vi "System Configuration_Generator.vi"() -> ()   [LabVIEW 2020]
uses:
  LabVIEW 2020 Toolkits/VI Server Toolkit/VI Server_TypeDefs/VI Server_RefsCluster.ctl
  LabVIEW 2020 Toolkits/toolkits_lv2020_32bit/Synchronization.llb/SynchRefs_SetGet.ctl
  LabVIEW 2020 Toolkits/VI Server Toolkit/VI Server Libraries/VI Server_GetControl.llb/VI Server_1D_Array_STR_Get.vi
  LabVIEW 2020 Toolkits/VI Server Toolkit/VI Server Toolkit LV2013.lvlib
panel:
  in  "TabControls.SAVE":bool
  in  "TabControls.Name":string[](array[string])=["Tab.Main"] caption="Target VI: Tab Control Names"
  in  "VI.Server.Port":u32=3363 caption="VI Server Port"
  in  "SystemSettings.SAVE":bool caption="TabControls.SAVE"
  in  "SAVE":bool
  in  "Generate":bool caption="Generate [SET]"
  in  "Ind.Symbols":i32[](array[numeric])
  in  "Ctl.Symbols":i32[](array[numeric])
  out "#OfIndicators":i32 caption="# Of Indicators"
  in  "Tab.Main":enum32{"CONTROLS", "DATA", "INDICATORS"}(tab)
  in  "Controls":i32[](listbox)
  in  "[SET]":string
  in  "[GET] ARGUMENT 2":u16(ring) caption="[GET] ARGUMENT 2 Prototype" items=["AI.Averaged.Mesurement", "AI.ActualSampleRate", "AO.ActualSampleRate", "DI.Port.Lines.0:7", "DI.Port.Lines.8:15", "DI.Port.Lines.16:23", "DI.Port.Lines.24:31", "DI.Line.State", "DO.Line.State.Verify", "DO.Port.State.Verify", "**********************", "ctr0.In.Count", "ctr0.Out.Frequency.Actual", "ctr0.Out.Duty Cycle.Actual", "ctr1.In.Count", "ctr2.In.Count", "ctr3.In.Count", "ctr1.Out.Frequency.Actual", "ctr1.Out.Duty Cycle.Actual", "ctr2.Out.Frequency.Actual", "ctr2.Out.Duty Cycle.Actual", "ctr3.Out.Frequency.Actual", "ctr3.Out.Duty Cycle.Actual"]
  in  "[SET] ARGUMENT 2":u16(ring) caption="[SET] ARGUMENT 2 Prototype" items=["AI.Sample.Mode", "AI.TerminalConfiguration", "AI.MaxInputLimit", "AI.MinInputLimit", "AI.SampleRate", "AI.Number.Of.Samples", "AI.Measure", "AI.PhysicalChannel.Include", "AI.MultiChannelAcquisition", "**********************", "AO.Output", "AO.MinVoltage", "AO.MaxVoltage", "AO.SampleRate", "AO.NumberOfSamples", "AO.GenerationMode", "AO.SinewaveFrequency", "AO.SampleMode", "AO.Update", "**********************", "DI.Line.Update", "DI.Port.Update", "DO.Line.Update", "DO.Port.Lines.7:0", "DO.Port.Lines.15:8", "DO.Port.Lines.23:16", "DO.Port.Lines.31:24", "DO.Port.Update", "DO.Line.State", "DO.Port.Lines.7:0.Mask", "DO.Port.Lines.15:8.Mask", "DO.Port.Lines.23:16.Mask", "DO.Port.Lines.31:24.Mask", "DO.Port.Mask.Apply", "**********************", "Cntr.In.ActiveEdge", "Cntr.In.IntegrationTime", "Cntr.In.Start", "Cntr.Out.Frequency", "Cntr.Out.Duty.Cycle", "Cntr.Out.Sample.Mode", "Cntr.Out.Start", "Cntr.Out.NumberOfPulses", "Settings.LOAD", "Settings.Name.New"]
  in  "[Argument 3: Data Type]":string
  in  "[GET]":string
  in  "Indicators":i32[](listbox)
  in  "EXIT":bool
  in  "DataSource.FileType":i32(ring) caption="Data Source: FileType" items=["VI", "File: *.cfg"]
  out "#OfControls":i32 caption="# Of Controls"
  in  "SoftPanel.V.Load":bool caption="Data Source: Load"
  in  "SoftPanel.VI.Path":path caption="Soft Panel VI  Path"
  out "error out":errorcluster
  in  "error in":errorcluster
  # "INSTRUCTIONS:\n1. Select Soft Panel VI and press the button \"LOAD\".\n2. On the [CONTROLS] page, table \"Controls\", by double click, mark indicators which will be excluded from \nbeing included into a System Configuration.cfg file of the soft panel. \n3. On the [INDICTORS] page, table \"Indicators\", by double click mark indicators which will be excluded from \nbeing included into a System Configuration.cfg file of the soft panel.\n4. Press the \"GENERATE\" button and examine data in the [SET], [Argument3: data Type], and [GET] tables.\n5. Press the \"SAVE\" button to transfer data to the System Configuration.cfg file."
  # "System Settings"
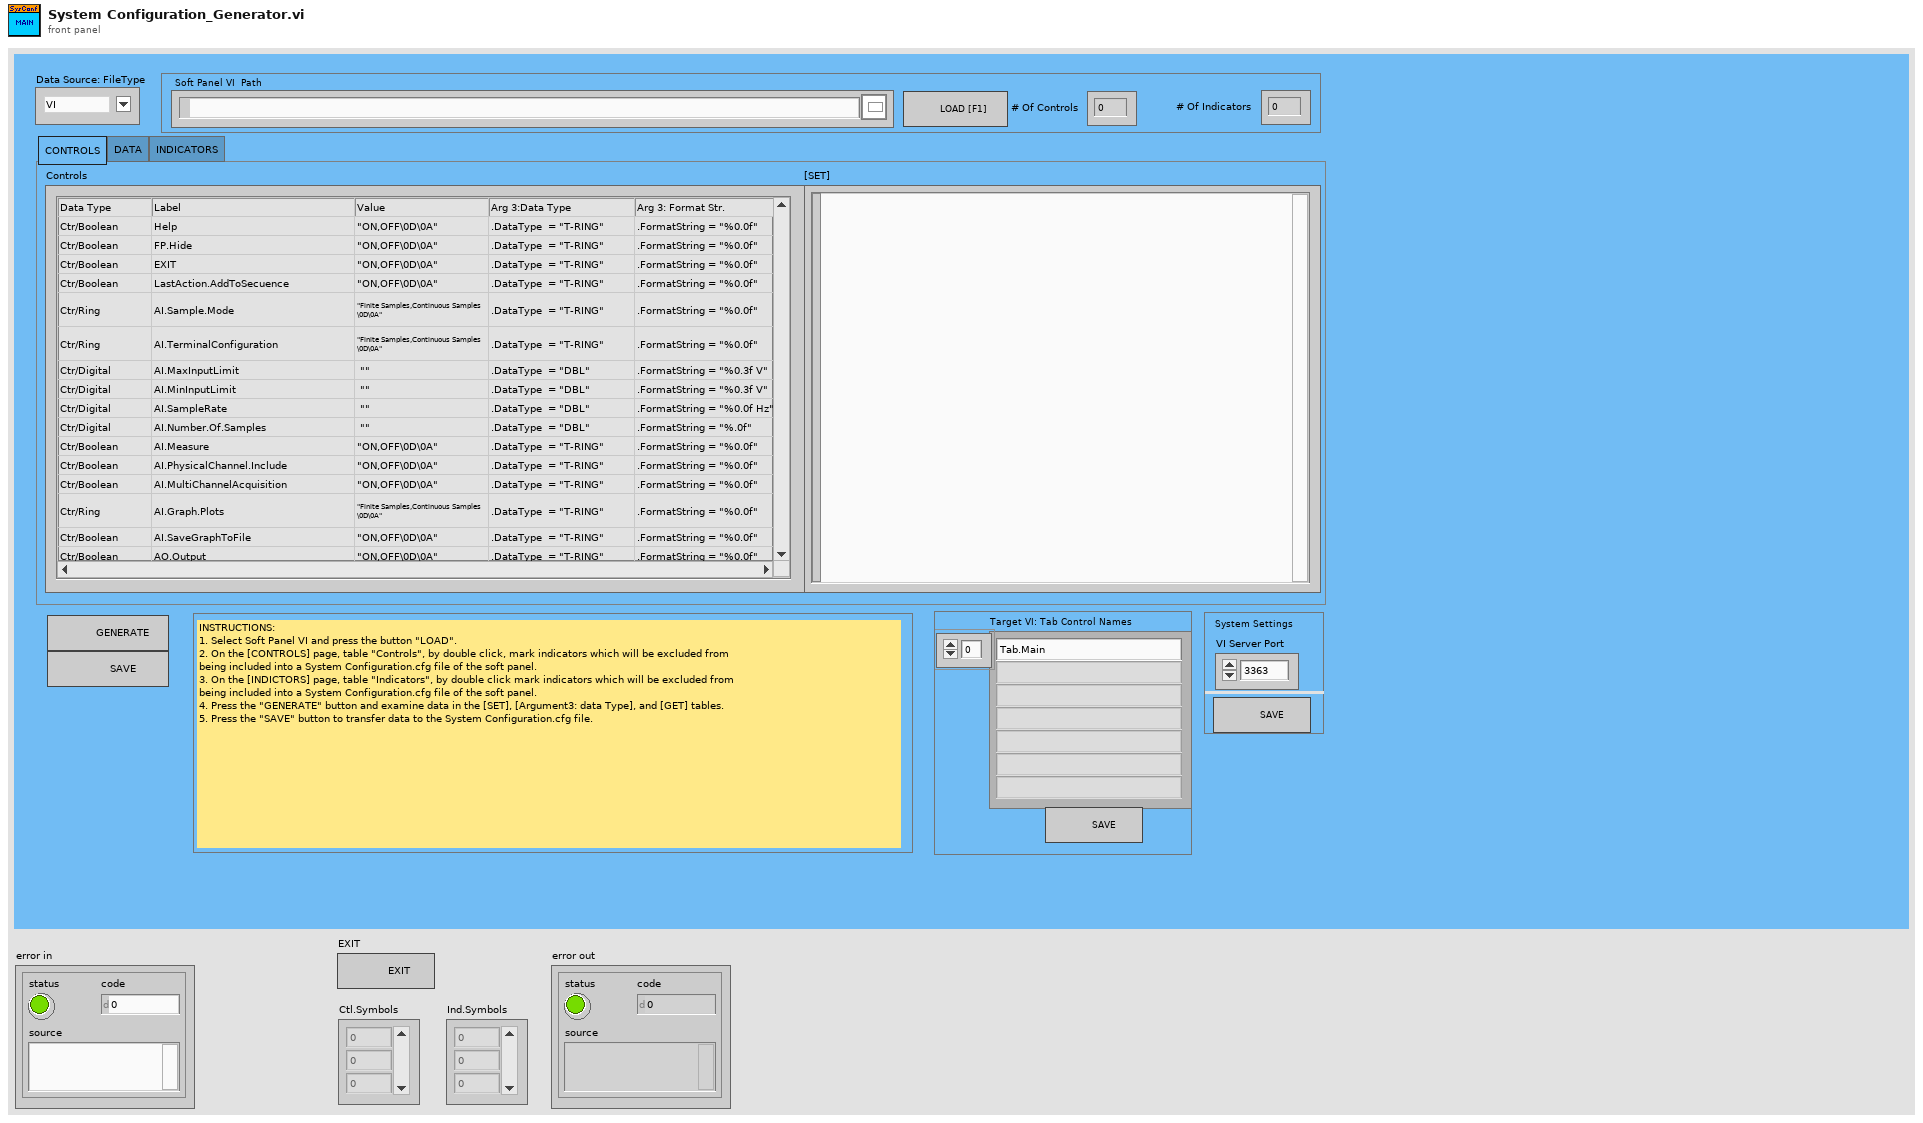
[diagram p1: front panel]
types:
  T1 = typedef "SynchRefs_SetGet.ctl" = enum16{"Set", "Get"}
  T2 = typedef "VI Server_RefsCluster.ctl" = cluster{"Labels":string[], "Refs":refnum<vi>[], "VI Ref":refnum<vi>}
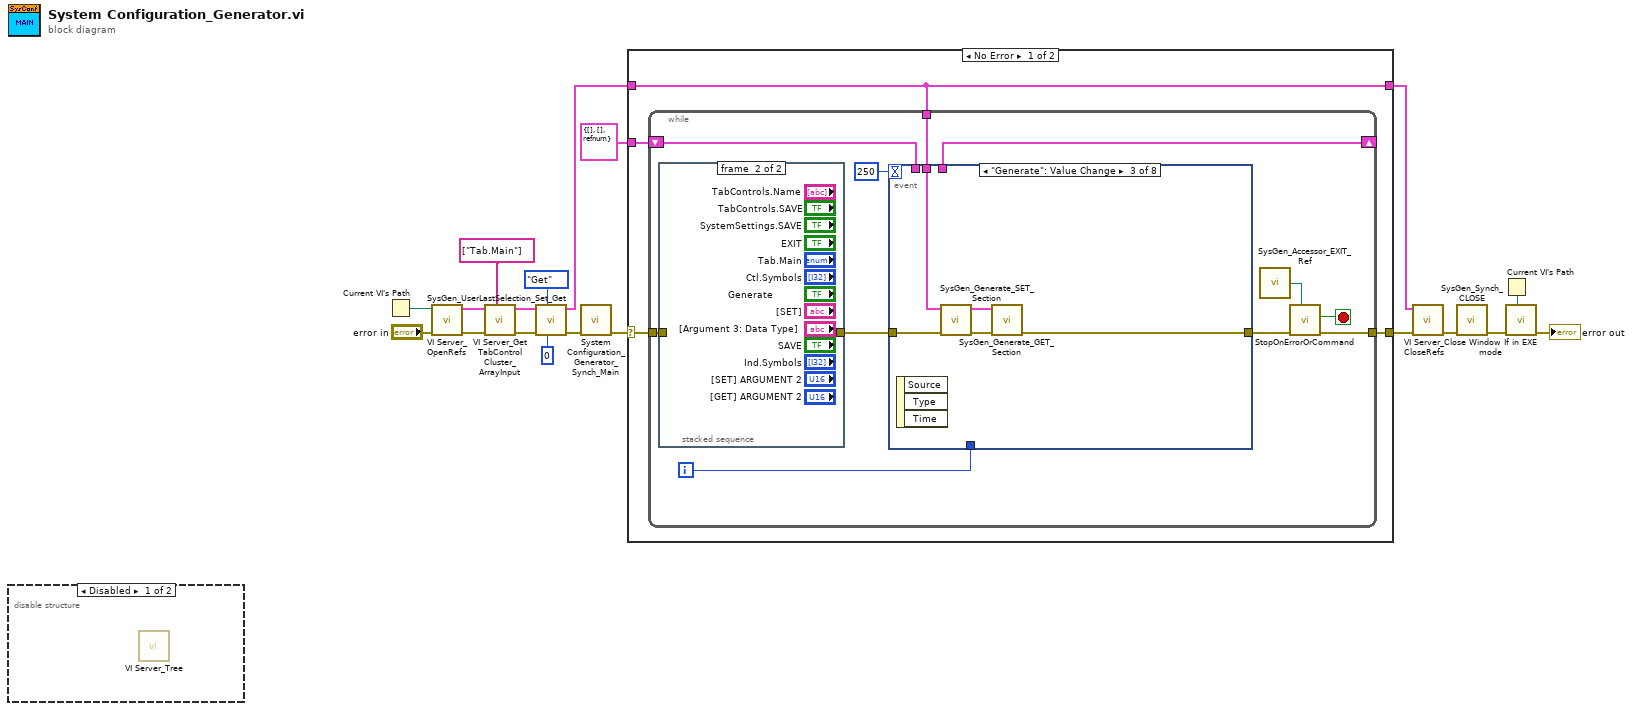
[diagram p0: block diagram]
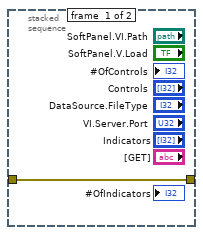
[diagram p2: hidden frame]
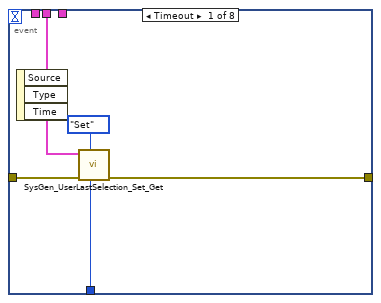
[diagram p3: hidden frame]
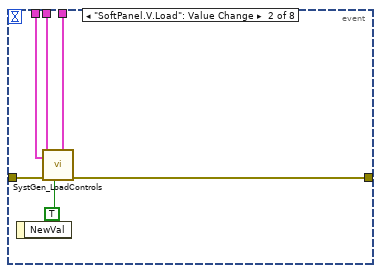
[diagram p4: hidden frame]
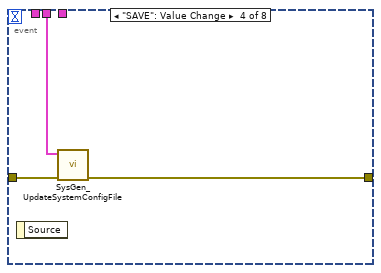
[diagram p5: hidden frame]
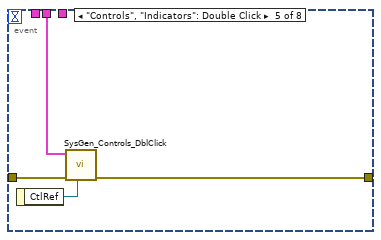
[diagram p6: hidden frame]
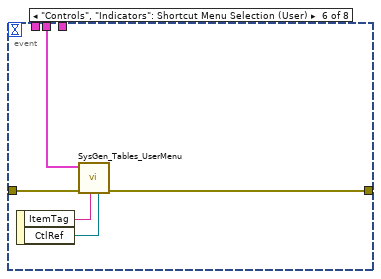
[diagram p7: hidden frame]
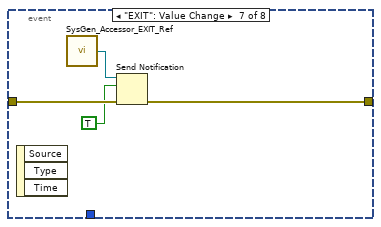
[diagram p8: hidden frame]
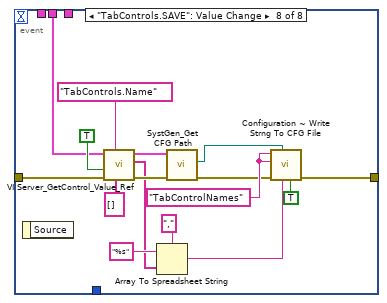
[diagram p9: hidden frame]
diagram:
  n1 = disable-structure shown="Disabled" {
    frame Disabled {
      n2 = call "VI Server_Tree.vi"() -> ()  [unwired: 12 in]
    }
    frame Enabled {
    }
  }
  n3 = Current VI's Path() -> (path=w18:path)
  n4 = call "VI Server_OpenRefs.vi"("error in"="error in", "VI Path"=w18) -> ("error out"=w6:errorcluster, "VI Server.RefsCluster"=w8:T2)  [unwired: 8 in]
  n5 = call "VI Server_Get TabControl Cluster_ArrayInput.vi"("TabControl Labels[]"=string[] ["Tab.Main"], "error in"=w6, "VI Server Cluster"=w8) -> ("error out"=w5:errorcluster, "VI Server Cluster.OUT"=w7:T2)  [unwired: 7 in]
  n6 = call "SysGen_UserLastSelection_Set_Get.vi"("LoopCounter"=0, "SynchRefs.Set/Get"=SynchRefs_SetGet."Get", "error in"=w5, "VI Server.RefsCluster"=w7) -> ("error out"=w13:errorcluster, "VI Server.RefsCluster.DUP"=w12:T2)  [unwired: 6 in]
  n7 = call "System Configuration_Generator_Synch_Main.vi"("error in"=w13) -> ("error out"=w16:errorcluster)  [unwired: 10 in]
  n8 = case shown="No Error" w16 {
    selector: w16 -> [w23 w85]
    tunnel: [w22 w85] -> w17
    tunnel: w12 -> [w21 w84]
    tunnel: [w21 w84] -> w14
    tunnel: T2 {"Labels"=[], "Refs"=[], "VI Ref"=refnum} ("VI ServerCluster DUP") -> [w20 _]
    frame No Error {
      n9 = while {
        tunnel: w23 -> [w34]
        tunnel: [w33] -> w22
        tunnel: w21 -> [w27]
        shift-right: [w24] -> _
        shift-left: w20 -> [w25]
        i -> [w26]
        stop <- w32 stop-if-true
        n10 = stacked-sequence {
          tunnel: w34 -> [w35 _]
          tunnel: [w35 _] -> w31
          frame #0 {
          }
          frame #1 {
          }
        }
        n11 = event shown="[2] \"Generate\": Value Change" {
          selector: _ -> [_ _ _ _ _ _ _ _]
          dyn-events: _ -> [_ _ _ _ _ _ _ _]
          timeout: 250 -> [_ _ _ _ _ _ _ _]
          tunnel: w31 -> [w40 w46 w51 w54 w58 w63 w67 w70]
          tunnel: [w36 w43 w48 w53 w56 w62 w66 w69] -> w30
          tunnel: w27 -> [w39 w45 w50 w52 w57 w59 _ w68]
          tunnel: w26 -> [w37 _ _ _ _ _ _ _]
          tunnel: w25 -> [_ w44 _ _ _ _ _ _]
          tunnel: [_ w42 _ _ _ _ _ _] -> w24
          event Timeout {
            n12 = event-data() -> ()  [unwired: 1 in, 3 out]
            n13 = call "SysGen_UserLastSelection_Set_Get.vi"("LoopCounter"=w37, "SynchRefs.Set/Get"=SynchRefs_SetGet."Set", "error in"=w40, "VI Server.RefsCluster"=w39) -> ("error out"=w36:errorcluster)  [unwired: 6 in, 1 out]
          }
          event "SoftPanel.V.Load": Value Change {
            n14 = event-data() -> ()  [unwired: 1 in, 1 out]
            n15 = call "SystGen_LoadControls.vi"("IgnoreClusters"=TRUE, "VI ServerCluster (Target VI)"=w44, "error in"=w46, "VI Server Cluster (Description VI)"=w45) -> ("error out"=w43:errorcluster, "VI ServerCluster (Target VI) OUT"=w42:T2)  [unwired: 5 in, 1 out]
          }
          event "Generate": Value Change {
            n16 = event-data() -> ()  [unwired: 1 in, 3 out]
            n17 = call "SysGen_Generate_SET_Section.vi"("error in (no error)"=w51, "VI Server.RefsCluster"=w50) -> ("error out"=w49:errorcluster, "VI Server Cluster.DUP"=w47:T2)  [unwired: 8 in]
            n18 = call "SysGen_Generate_GET_Section.vi"("error in (no error)"=w49, "VI Server.RefsCluster"=w47) -> ("error out"=w48:errorcluster)  [unwired: 8 in, 1 out]
          }
          event "SAVE": Value Change {
            n19 = event-data() -> ()  [unwired: 1 in, 1 out]
            n20 = call "SysGen_UpdateSystemConfigFile.vi"("error in (no error)"=w54, "VI Server.RefsCluster"=w52) -> ("error out"=w53:errorcluster)  [unwired: 9 in]
          }
          event "Controls", "Indicators": Double Click {
            n21 = event-data() -> ("CtlRef"=w55:refnum<vi>)  [unwired: 1 in]
            n22 = call "SysGen_Controls_DblClick.vi"("CtlRef"=w55, "error in (no error)"=w58, "VI Server.RefsCluster"=w57) -> ("error out"=w56:errorcluster)  [unwired: 8 in]
          }
          event "Controls", "Indicators": Shortcut Menu Selection (User) {
            n23 = event-data() -> ("ItemTag"=w61:string, "CtlRef"=w60:refnum<vi>)  [unwired: 1 in]
            n24 = call "SysGen_Tables_UserMenu.vi"("MulticolumnListbox in"=w60, "ItemTag"=w61, "error in (no error)"=w63, "VI Server.RefsCluster"=w59) -> ("error out"=w62:errorcluster)  [unwired: 7 in]
          }
          event "EXIT": Value Change {
            n25 = event-data() -> ()  [unwired: 1 in, 3 out]
            n26 = call "SysGen_Accessor_EXIT_Ref.vi"() -> ("EXIT"=w65:refnum<notifier>)  [unwired: 6 in]
            n27 = Send Notification(notification=TRUE, notifier=w65, error in (no error)=w67) -> (error out=w66:errorcluster)  [unwired: 1 out]
          }
          event "TabControls.SAVE": Value Change {
            w81 = "TabControlNames" ("key")
            n28 = event-data() -> ()  [unwired: 1 in, 1 out]
            n29 = call-poly "VI Server_GetControl_Value_Ref.vi"("DataType"=string[] [], "Control.Label"="TabControls.Name" ("Label"), "error in"=w70, "SingleInstance"=TRUE ("Single Instance (T)"), "VI Server.RefsCluster"=w68) -> ("error out"=w77:errorcluster, "Value"=w73:string[], "VI Server.RefsCluster.DUP"=w78:T2)  [unwired: 3 in, 1 out]
            n30 = Array To Spreadsheet String(delimiter (Tab)=",", array=w73, 3:"%s" ("format string")) -> (spreadsheet string=w76:string)
            n31 = call "SystGen_Get CFG Path.vi"("error in"=w77, "VI Server Cluster"=w78) -> ("error out"=w79:errorcluster, "CFG File  path"=w80:path)  [unwired: 6 in, 2 out]
            n32 = call "Configuration ~ Write Strng To CFG File.vi"("CloseFIle"=TRUE, "String"=w76, "configuration file path"=w80, "error in (no error)"=w79, "Key"=w81, "section"=w81) -> ("error out"=w69:errorcluster)  [unwired: 4 in, 1 out]
          }
        }
        n33 = call "SysGen_Accessor_EXIT_Ref.vi"() -> ("EXIT"=w28:refnum<notifier>)  [unwired: 6 in]
        n34 = call "StopOnErrorOrCommand.vi"("STOP"=w28, "error in (no error)"=w30) -> ("error out"=w33:errorcluster, "STOP"=w32:bool)  [unwired: 8 in]
      }
    }
    frame Error {
    }
  }
  n35 = call "VI Server_CloseRefs.vi"("error in"=w17, "VI Server.RefsCluster"=w14) -> ("error out"=w15:errorcluster)  [unwired: 9 in]
  n36 = call "SysGen_Synch_CLOSE.vi"("error in"=w15) -> ("error out"=w2:errorcluster)  [unwired: 10 in]
  n37 = Current VI's Path() -> (path=w3:path)
  n38 = call "Close Window If in EXE mode.vi"("TopLevelVI Path"=w3, "error in"=w2) -> ("error out"=→"error out":errorcluster)  [unwired: 9 in]
